vi "Configure Current Limit.vi"(7 "Behavior (0: Regulate)":u16(ring) items=["Regulate", "Trip"], 8 "error in (no error)":errorcluster, 9 "Current Limit (5.0 A)":dbl=5.0 caption="Current Limit (5 A)" format="%.2f", 10 "Channel (0: +6V Channel)":i32(ring) caption="Channel (0: +6V)" items=["+6V Channel", "+25V Channel", "-25V Channel"], 11 "VISA resource name":refnum<visa-resource-name>) -> (0 "error out":errorcluster, 3 "VISA resource name out":refnum<visa-resource-name>)   [LabVIEW 2020, in "RIGOL DP1000 Series.lvlib"]
doc: "Configures over current protection (OCP). Specify the output current limit value and the behavior of the power supply when the output current is greater than or equal to that value."
uses:
  <instrlib>/RIGOL DP1000 Series/RIGOL DP1000 Series.lvlib
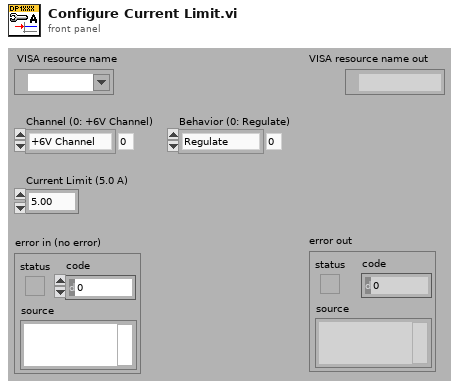
[diagram p1: front panel]
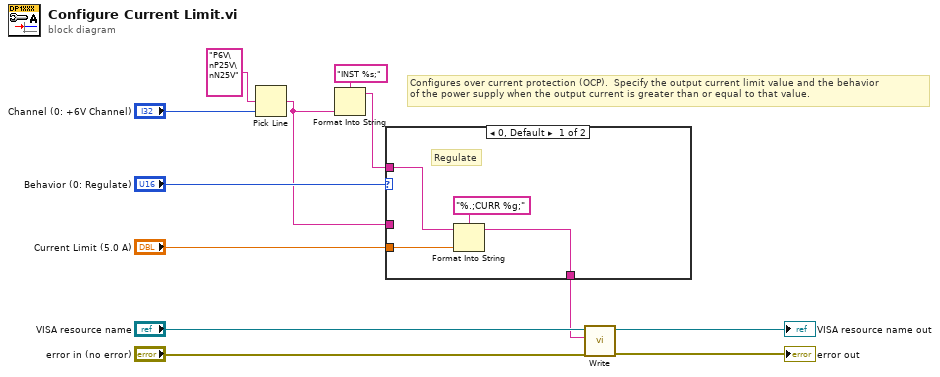
[diagram p0: block diagram]
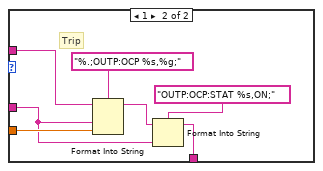
[diagram p2: hidden frame]
diagram:
  # "Configures over current protection (OCP).  Specify the output current limit value and the behavior \nof the power supply when the output current is greater than or equal to that value."
  n1 = Pick Line(multi-line string="P6V\nP25V\nN25V", line index="Channel (0: +6V Channel)") -> (output string=w6:string)  [unwired: 1 in]
  n2 = Format Into String(format string="INST %s;", w6) -> (resulting string=w8:string)  [unwired: 2 in, 1 out]
  n3 = case shown="0, Default" "Behavior (0: Regulate)" {
    tunnel: "Current Limit (5.0 A)" -> [w15 w22]
    tunnel: w8 -> [w14 w21]
    tunnel: [w13 w19] -> w1
    tunnel: w6 -> [_ w18]
    frame 0, Default {
      # "Regulate"
      n4 = Format Into String(format string="%.;CURR %g;", initial string=w14, w15) -> (resulting string=w13:string)  [unwired: 1 in, 1 out]
    }
    frame 1 {
      # "Trip"
      n5 = Format Into String(format string="%.;OUTP:OCP %s,%g;", initial string=w21, w18, w22) -> (resulting string=w20:string)  [unwired: 1 in, 1 out]
      n6 = Format Into String(format string="OUTP:OCP:STAT %s,ON;", initial string=w20, w18) -> (resulting string=w19:string)  [unwired: 1 in, 1 out]
    }
  }
  n7 = call <instrlib>:"Write.vi"("error in (no error)"="error in (no error)", "Write Buffer (\"\")"=w1, "VISA resource name"="VISA resource name") -> ("error out"=→"error out":errorcluster, "VISA resource name out"=→"VISA resource name out":refnum<visa-resource-name>)  [unwired: 7 in]
